vi "read LUA Table.vi"(8 "error in (no error)":errorcluster, 10 "vali_or_spec":string, 11 "filename":string) -> (0 "error out":errorcluster, 3 "function return":bool)   [LabVIEW 2019, in "libSpecValiReader.lvlib"]
doc: "bool readLUATable(const char* filename, const char* vali_or_spec);"
uses:
  libSpecValiReader.lvlib
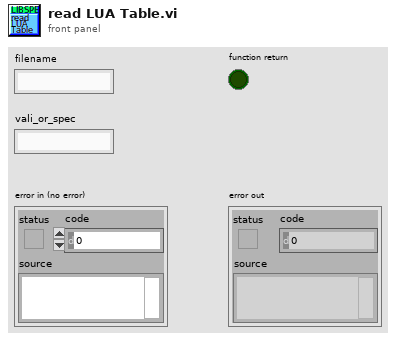
[diagram p1: front panel]
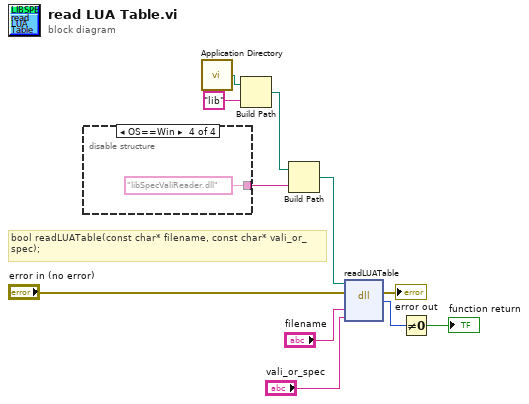
[diagram p0: block diagram]
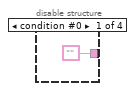
[diagram p2: hidden frame]
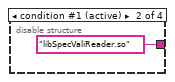
[diagram p3: hidden frame]
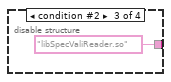
[diagram p4: hidden frame]
diagram:
  # "bool readLUATable(const char* filename, const char* vali_or_spec);"
  n1 = disable-structure shown="OS==Win" {
    disable-tunnel: ["" "libSpecValiReader.so" ("name or relative path") "libSpecValiReader.so" ("name or relative path") "libSpecValiReader.dll" ("name or relative path")] -> w2
    frame condition #0 {
    }
    frame condition #1 (active) {
    }
    frame condition #2 {
    }
    frame condition #3 {
    }
  }
  n2 = call <vilib>:"Application Directory.vi"() -> ("Application Directory"=w5:path)
  n3 = Build Path(base path=w5, name or relative path="lib") -> (appended path=w3:path)
  n4 = Build Path(base path=w3, name or relative path=w2) -> (appended path=w1:path)
  n5 = dll-call lib="home/paul/Schreibtisch/Biogas_plant_setup/LabView/lib/libSpecValiReader/libSpecValiReader.*" fn="readLUATable"(path in=w1, error in="error in (no error)", "filename"="filename", "vali_or_spec"="vali_or_spec") -> (error out=→"error out":errorcluster, "return type"=w10:u8)  [unwired: 3 in, 1 out]
  n6 = Not Equal To 0?(x=w10) -> (x != 0?=→"function return":bool)
